vi "Launch Nested Actor Friend Wrapper.vi"(4 "Debug Alias":string, 6 "Open Actor Core front panel? (F)":bool, 8 "error in (no error)":errorcluster, 9 "Auto-stop? (T)":bool=TRUE, 10 "Nested Actor":refnum<class "Actor.lvclass">, 11 "Caller Actor in":refnum<class "Actor.lvclass">) -> (0 "error out":errorcluster, 2 "Nested Actor's Enqueuer":refnum<class "Message Enqueuer.lvclass">, 3 "Caller Actor out":refnum<class "Actor.lvclass">)   [LabVIEW 2020, in "Actor Framework.lvlib" / "Actor.lvclass"]
doc: "(<B>Filename</B>: Actor Framework.lvlib:Actor.lvclass:Launch Nested Actor Friend Wrapper.vi)\n\nThis VI is a community-scoped wrapper around Actor Framework.lvlib:Actor.lvclass:Launch Nested Actor.vi. It is a behind-the-scenes component of the Actor Framework."
uses:
  <vilib>/ActorFramework/Actor/Actor.lvclass
  <vilib>/ActorFramework/Message Enqueuer/Message Enqueuer.lvclass
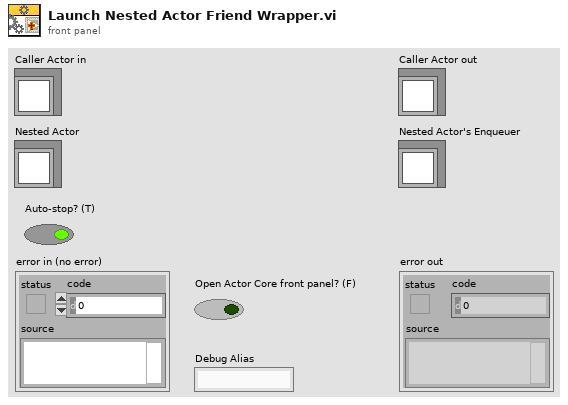
[diagram p1: front panel]
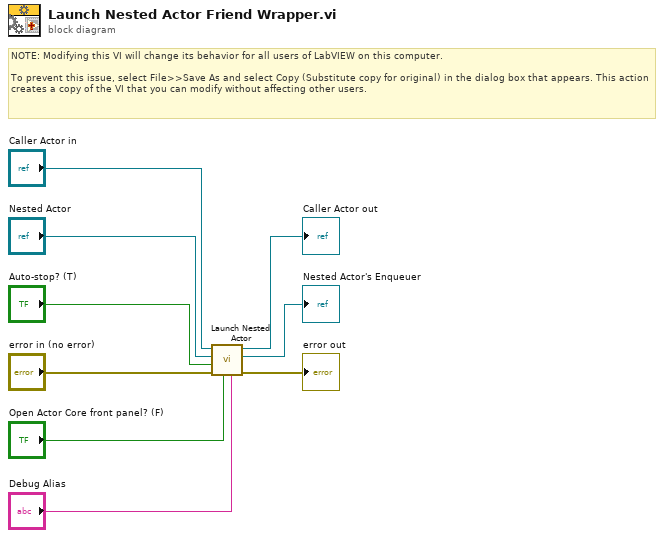
[diagram p0: block diagram]
diagram:
  # "NOTE: Modifying this VI will change its behavior for all users of LabVIEW on this computer.\n\nTo prevent this issue, select File>>Save As and select Copy (Substitute copy for original) in the dialog box that appears. This action creates a copy of the VI that you can modify without affecting other users."
  n1 = call <vilib>:"Launch Nested Actor.vi"("Debug Alias"="Debug Alias", "Open Actor Core front panel? (F)"="Open Actor Core front panel? (F)", "error in (no error)"="error in (no error)", "Auto-stop? (T)"="Auto-stop? (T)", "Nested Actor"="Nested Actor", "Caller Actor in"="Caller Actor in") -> ("error out"=→"error out":errorcluster, "Nested Actor's Enqueuer"=→"Nested Actor's Enqueuer":refnum<class "Message Enqueuer.lvclass">, "Caller Actor out"=→"Caller Actor out":refnum<class "Actor.lvclass">)  [unwired: 3 in]
